vi "_dummy4_.vi"() -> ()   [LabVIEW 2017, in "_dummy3_.lvclass"]
uses:
  _dummy3_.lvclass
panel:
  out "DUMMY METHOD":bool
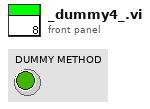
[diagram p1: front panel]
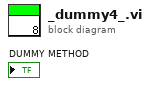
[diagram p0: block diagram]
diagram:
